vi "Binary_SpectroscopyFile-ProcessTemplate.vi"(6 "Config":T1, 8 "error in (no error)":errorcluster, 9 "data":sgl[][](array[numeric]) format="%#_4p", 10 "Parameter values":sgl[](array[numeric]) format="%#_6p", 11 "Configuration":T2={"Mode"=enum."dI/dV @ V", "Bias voltage"=0.0, "Window width\n(# Points for fit)"=5, "Polynomial order\n(I/V @ V only)"=3}) -> (0 "error out":errorcluster, 3 "Output value":sgl)   [LabVIEW 2017]
uses:
  Nanonis Prog Interface.lvlib
  <vilib>/Analysis/NI_AALPro.lvlib
  File/Binary_SpectroscopyFile-Config.ctl
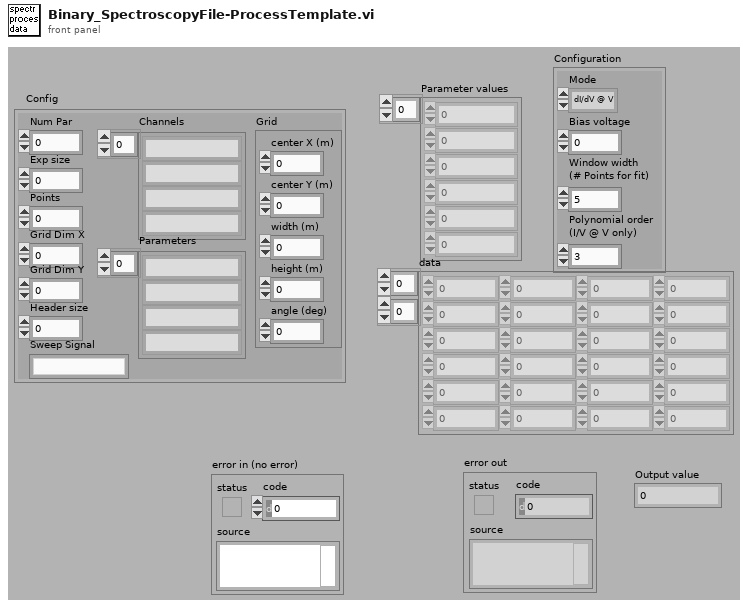
[diagram p1: front panel]
types:
  T1 = typedef "Nanonis Prog Interface.lvlib/Binary_SpectroscopyFile-Config.ctl" = cluster{"Num Par":i32, "Exp size":i32, "Points":i32, "Grid Dim X":i32, "Grid Dim Y":i32, "Header size":i32, "Channels":string[], "Parameters":string[], "Sweep Signal":string, "Grid":cluster{"center X (m)":sgl, "center Y (m)":sgl, "width (m)":sgl, "height (m)":sgl, "angle (deg)":sgl}}
  T2 = cluster{"Mode":enum16{"I @ V", "dI/dV @ V"}, "Bias voltage":sgl, "Window width\n(# Points for fit)":i32, "Polynomial order\n(I/V @ V only)":i32}
  T3 = enum32{"SVD", "Givens", "Givens2", "Householder", "LU Decomposition", "Cholesky"}
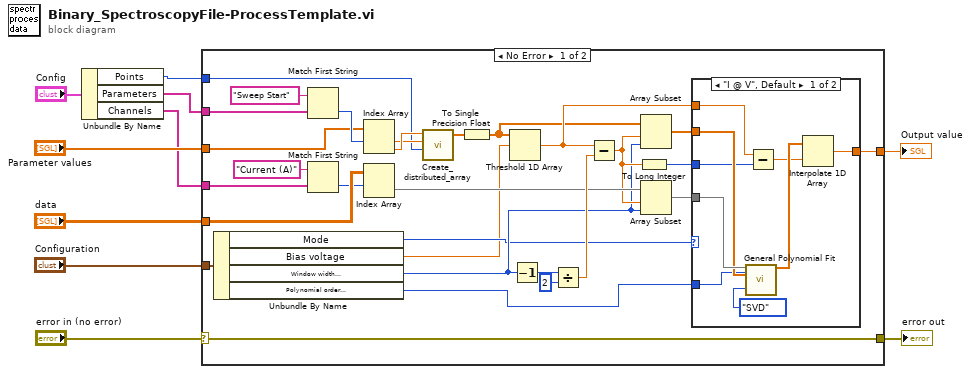
[diagram p0: block diagram]
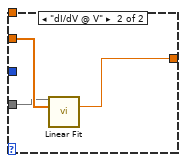
[diagram p2: hidden frame]
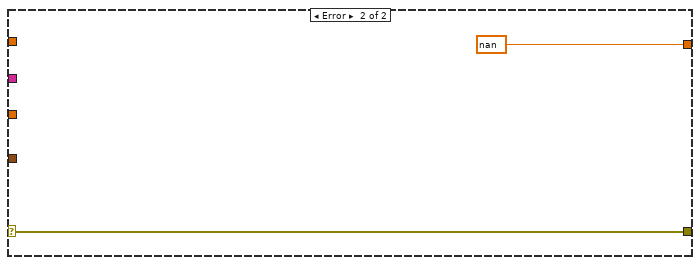
[diagram p3: hidden frame]
diagram:
  n1 = Unbundle By Name("Config") -> ("Points"=w2:i32, "Parameters"=w4:string[], "Channels"=w3:string[])
  n2 = case shown="No Error" "error in (no error)" {
    selector: "error in (no error)" -> [w39 w53]
    tunnel: [w39 w53] -> w9
    tunnel: w4 -> [w17 _]
    tunnel: "Parameter values" -> [w16 _]
    tunnel: w3 -> [w36 _]
    tunnel: "data" -> [w34 _]
    tunnel: [w23 sgl nan ("element")] -> w6
    tunnel: "Configuration" -> [w22 _]
    tunnel: w2 -> [w11 _]
    frame No Error {
      n3 = Unbundle By Name(w22) -> ("Mode"=w19:enum16{"I @ V", "dI/dV @ V"}, "Bias voltage"=w18:sgl, "Window width\n(# Points for fit)"=w21:i32, "Polynomial order\n(I/V @ V only)"=w20:i32)
      n4 = Match First String(2:w17, 3:"Sweep Start" ("string")) -> (0:w35:i32)  [unwired: 1 out]
      n5 = Match First String(2:w36, 3:"Current (A)" ("string")) -> (0:w33:i32)  [unwired: 1 out]
      n6 = Index Array(array=w16, index #1=w35) -> (element #1=w13:sgl, element #2=w14:sgl)  [unwired: 1 in]
      n7 = Index Array(array=w34, index (row)=w33) -> (element=w29:sgl[])  [unwired: 1 in]
      n8 = call "Create_distributed_array.vi"("Upper Lim"=w14, "Lower Lim"=w13, "Num Points"=w11) -> ("Array"=w15:dbl[])  [unwired: 3 in]
      n9 = To Single Precision Float(number=w15) -> (single precision float=w12:sgl[])
      n10 = Threshold 1D Array(2:w18, 3:w12) -> (0:w26:sgl)  [unwired: 1 in]
      n11 = Decrement(x=w21) -> (x-1=w32:i32)
      n12 = Divide(x=w32, y=2) -> (x/y=w30:dbl)
      n13 = Subtract(x=w26, y=w30) -> (x-y=w25:dbl)
      n14 = To Long Integer(number=w25) -> (32bit integer=w24:i32)
      n15 = Array Subset(array=w12, index=w25, length=w21) -> (w27:sgl[])
      n16 = Array Subset(array=w29, index=w25, length=w21) -> (w28:sgl[])
      n17 = case shown="\"I @ V\", Default" w19 {
        tunnel: w28 -> [w47 w50]
        tunnel: w27 -> [w46 w51]
        tunnel: w20 -> [w45 _]
        tunnel: w26 -> [w43 _]
        tunnel: w24 -> [w42 _]
        tunnel: [w40 w49] -> w23
        frame "I @ V", Default {
          n18 = call <vilib>:"General Polynomial Fit.vi"("Y"=w47, "polynomial order"=w45, "X"=w46, "algorithm"=T3."SVD") -> ("Best Polynomial Fit"=w44:dbl[])  [unwired: 8 in, 3 out]
          n19 = Subtract(x=w43, y=w42) -> (x-y=w41:sgl)
          n20 = Interpolate 1D Array(1:w41, 2:w44) -> (0:w40:dbl)
        }
        frame "dI/dV @ V" {
          n21 = call <vilib>:"Linear Fit.vi"("Y"=w50, "X"=w51) -> ("slope"=w49:dbl)  [unwired: 9 in, 4 out]
        }
      }
    }
    frame Error {
    }
  }
  "error out" <- w9
  "Output value" <- w6
